vi "SWRTIGEventListener.vi"(8 "error in":errorcluster, 11 "StellarNet Black-Comet Spec in":refnum<class "StellarNet Black-Comet Spec.lvclass">) -> (0 "error out":errorcluster, 2 "Triggered?":bool, 3 "StellarNet Black-Comet Spec out":refnum<class "StellarNet Black-Comet Spec.lvclass">)   [LabVIEW 2013, in "StellarNet Black-Comet Spec.lvclass"]
uses:
  StellarNet Black-Comet Spec.lvclass
  StellarNet Black-Comet Spec.lvclass/StellarNet Black-Comet Spec.ctl
  shared/GlobalVariables/SWTrigEventReference.vi
panel:
  in  "OK Button":bool
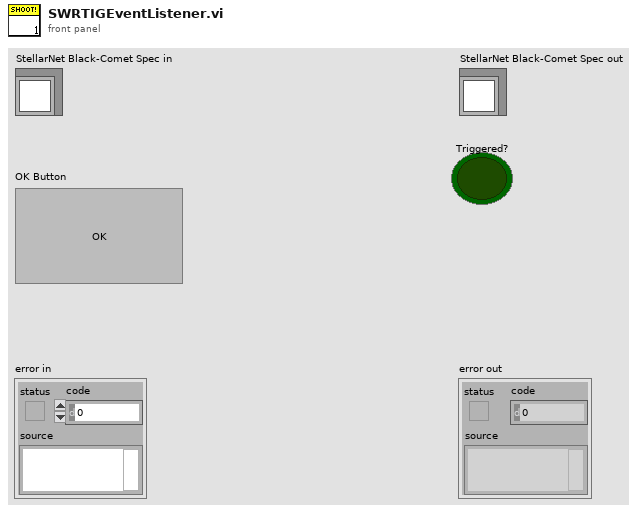
[diagram p1: front panel]
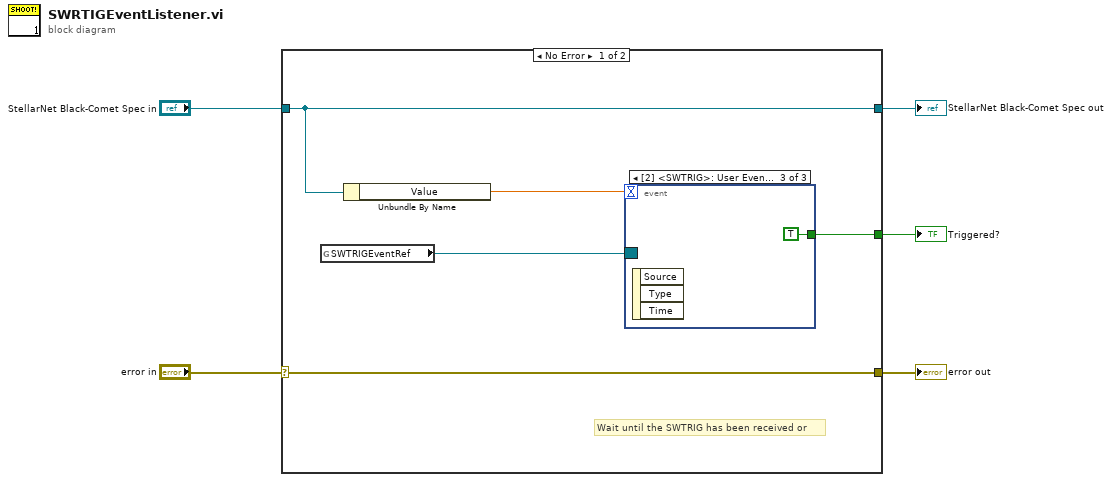
[diagram p0: block diagram]
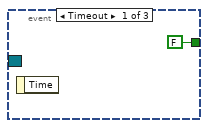
[diagram p2: hidden frame]
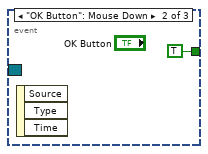
[diagram p3: hidden frame]
diagram:
  n1 = case shown="No Error" "error in" {
    selector: "error in" -> [w9 w15]
    tunnel: [w9 w15] -> w4
    tunnel: [w8 w14] -> w2
    tunnel: "StellarNet Black-Comet Spec in" -> [w8 w14]
    tunnel: [w10 _] -> w1
    frame No Error {
      # "Wait until the SWTRIG has been received or"
      n2 = global read "SWTrigEventReference.vi" "SWTRIGEventRef"() -> (w7:refnum<event-registration>)
      n3 = Unbundle By Name(w8) -> ("Value"=w6:dbl)
      n4 = event shown="[2] <SWTRIG>: User Event" {
        selector: w7 -> [_ _ _]
        dyn-events: _ -> [_ _ _]
        timeout: w6 -> [_ _ _]
        tunnel: [FALSE TRUE TRUE] -> w10
        event Timeout {
          n5 = event-data() -> ()  [unwired: 1 in, 1 out]
        }
        event "OK Button": Mouse Down {
          n6 = event-data() -> ()  [unwired: 1 in, 3 out]
        }
        event User Event {
          n7 = event-data() -> ()  [unwired: 1 in, 3 out]
        }
      }
    }
    frame Error {
    }
  }
  "error out" <- w4
  "StellarNet Black-Comet Spec out" <- w2
  "Triggered?" <- w1
